vi "Write to Port.vi"(8 "error in":errorcluster, 9 "Input Value":dbl, 10 "TEC Cmd":T1, 11 "TE Cooler in":refnum<class "TE Cooler.lvclass">) -> (0 "error out":errorcluster, 2 "String":string, 3 "TE Cooler out":refnum<class "TE Cooler.lvclass">)   [LabVIEW 2015, in "TE Cooler.lvlib" / "TE Cooler.lvclass"]
uses:
  TE Cooler.lvclass
  Controls/Command.ctl
  <vilib>/MSR Consulting, LLC/Devices/Configurable Device/Configurable Device.lvclass/Configurable Device.ctl
  <vilib>/MSR Consulting, LLC/Devices/Configurable Device/Accessors/Read Addr.vi
  <vilib>/MSR Consulting, LLC/Devices/Configurable Device/Read Log Session.vi
  <vilib>/MSR Consulting, LLC/General Reuse/Session APIs/_Session Fwk/Session - Root.lvclass
  <vilib>/MSR Consulting, LLC/General Reuse/Session APIs/Session Log/System Log.lvclass
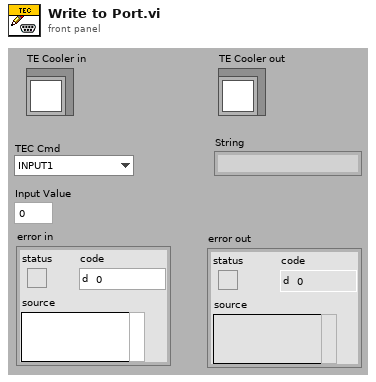
[diagram p1: front panel]
types:
  T1 = typedef "TE Cooler.lvlib/TE Cooler.lvclass/Command.ctl" = enum16{"INPUT1", "DESIRED CONTROL VALUE", "POWER OUTPUT", "ALARM STATUS", "INPUT 2", "OUTPUT CURRENT COUNTS", "ALARM TYPE", "SET TYPE DEFINE", "SENSOR TYPE", "CONTROL TYPE", "CONTROL OUTPUT POLARITY", "POWER ON/OFF", "OUTPUT SHUTDOWN IF ALARM", "FIXED DESIRED CONTROL SETTING", "PROPORTIONAL BANDWIDTH", "INTEGRAL GAIN", "DERIVATIVE GAIN", "LOW EXTERNAL SET RANGE", "HIGH EXTERNAL SET RANGE", "ALARM DEADBAND", "HIGH ALARM SETTING", "LOW ALARM SETTING", "CONTROL DEADBAND SETTING", "INPUT1 OFFSET", "INPUT2 OFFSET", "HEAT MULTIPLIER", "COOL MULTIPLIER", "OVER CURRENT COUNT COMPARE VALUE", "ALARM LATCH ENABLE", "NOT USED", "ALARM LATCH RESET", "CHOOSE SENSOR FOR ALARM FUNCTION", "CHOOSE TEMPERATURE WORKING UNITS", "EEPROM WRITE ENABLE", "OVER CURRENT CONTINUOUS", "OVER CURRENT RESTART ATTEMPTS", "JP3 DISPLAY ENABLE"}
  T2 = typedef "Session - Root.lvclass/Session Handle.ctl" = refnum<data-value>
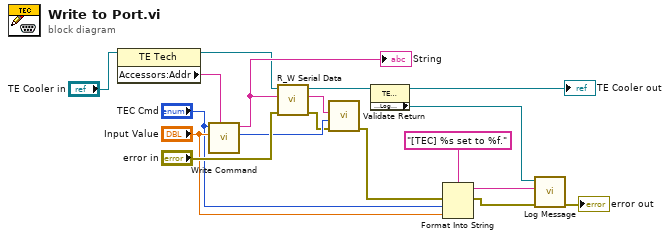
[diagram p0: block diagram]
diagram:
  n1 = property class="TE Tech"(reference="TE Cooler in") -> (reference out=w1:refnum<class "TE Cooler.lvclass">, "Accessors:Addr"=w2:string)  [unwired: 1 in, 1 out]
  n2 = call "Write Command.vi"("Addr"=w2, "Input Value"="Input Value", "TEC Cmd"="TEC Cmd") -> ("Divisor"=w16:i32, "Cmd"=w17:string)  [unwired: 7 in]
  "String" <- w17
  n3 = call "R_W Serial Data.vi"("error in"="error in", "String In"=w17, "TE Cooler in"=w1) -> ("error out"=w15:errorcluster, "String Out"=w14:string, "TE Cooler out"=w12:refnum<class "TE Cooler.lvclass">)  [unwired: 6 in]
  n4 = call "Validate Return.vi"("error in"=w15, "Divisor"=w16, "Rtn Str"=w14) -> ("error out"=w9:errorcluster)  [unwired: 6 in, 2 out]
  n5 = property class="TE Tech"(reference=w12) -> (reference out=→"TE Cooler out":refnum<class "TE Cooler.lvclass">, "Accessors:Log Session"=w13:T2)  [unwired: 1 in, 1 out]
  n6 = Format Into String(format string="[TEC] %s set to %f." ("Message In"), error in=w9, "TEC Cmd", "Input Value") -> (resulting string=w7:string, error out=w8:errorcluster)  [unwired: 1 in]
  n7 = call <vilib>:"Log Message.vi"("error in"=w8, "MSG In"=w7, "session in"=w13) -> ("error out"=→"error out":errorcluster)  [unwired: 7 in, 1 out]
